vi "TCP Vision - Receiver.vi"() -> ()   [LabVIEW 2019]
doc: "The UDP protocol differs from TCP in that there is no error-checking with the packets of information that are sent, and thus no guarantee whatsoever that an intended recipient will actually receive a given piece of data.\n\nUDP does offer the ability to \"broadcast\" data across a network--simply specify an IP Address of all ones (255.255.255.255) to attempt to broadcast information network-wide. Keep in mind that routers and other network hardware will generally refuse to forward the broadcast beyond certain points, so the extent of the broadcast will in practice be limited."
uses:
  UDP Main States.ctl
  <vilib>/vision/Image Controls.llb/IMAQ Image.ctl
panel:
  in  "receiver port":u16=1180
  out "Image":T1(plugin-control)
  out "error out":errorcluster
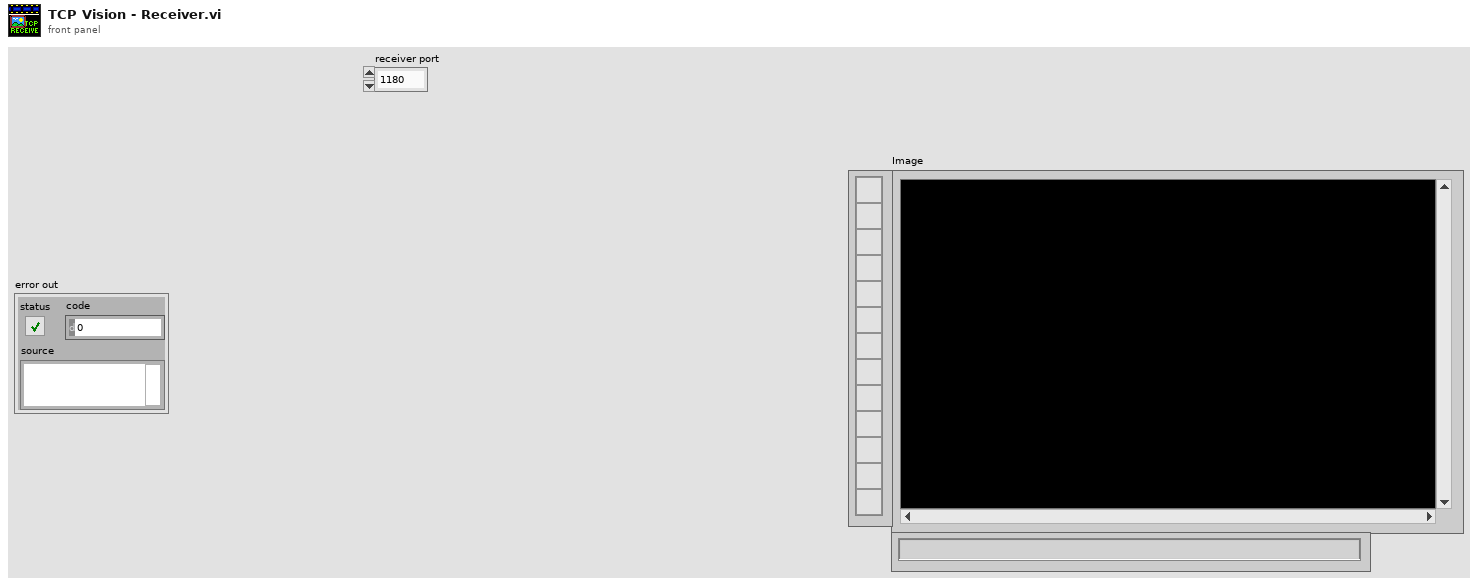
[diagram p1: front panel]
types:
  T1 = typedef "IMAQ Image.ctl" = refnum<image>
  T2 = typedef "UDP Main States.ctl" = enum16{"Message Dispatcher", "INI", "Read Data", "Send Data", "TCP Close", "TCP Open", "Exit"}
  T3 = enum16{"Standard", "Buffered", "CRLF", "Immediate"}
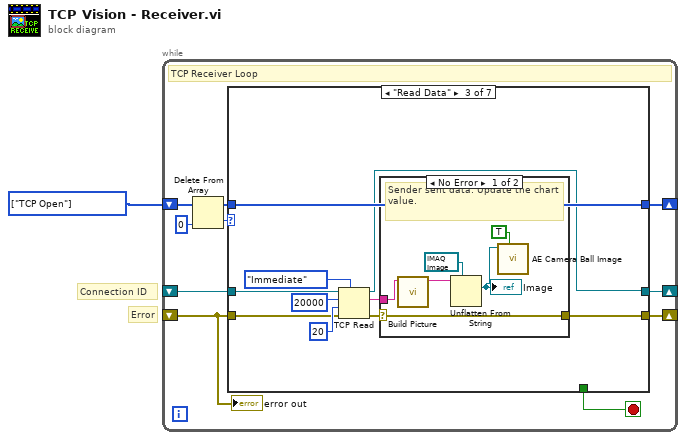
[diagram p0: block diagram]
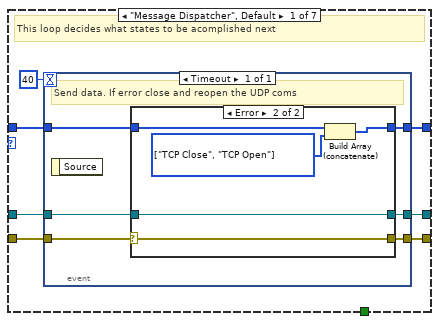
[diagram p2: hidden frame]
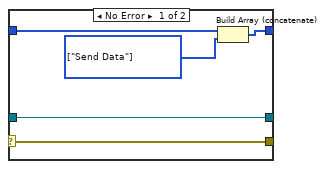
[diagram p3: hidden frame]
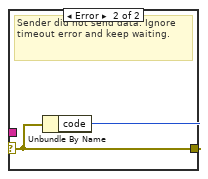
[diagram p5: hidden frame]
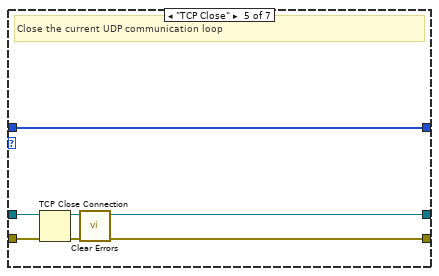
[diagram p8: hidden frame]
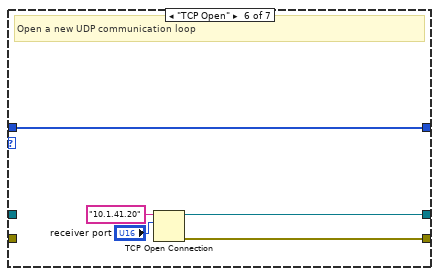
[diagram p9: hidden frame]
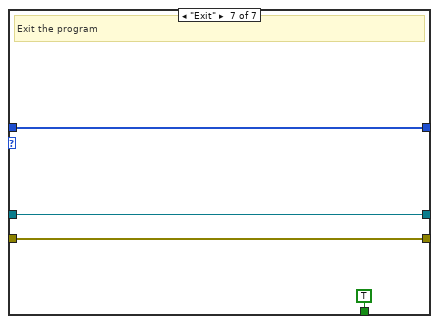
[diagram p10: hidden frame]
diagram:
  w1 = T2[] [enum."TCP Open"] items=["Message Dispatcher", "INI", "Read Data", "Send Data", "TCP Close", "TCP Open", "Exit"]
  # "Error"
  # "Connection ID"
  n1 = while {
    shift-right: [w3] -> _
    shift-left: w1 -> [w7]
    shift-right: [w11] -> _
    shift-left: _ -> [w9]
    shift-right: [w10] -> _
    shift-left: _ -> [w8]
    stop <- w2 stop-if-true
    # "TCP Receiver Loop"
    n2 = Delete From Array(array=w7, index=0) -> (deleted portion=w5:T2, array with subset deleted=w4:T2[])  [unwired: 1 in]
    n3 = case shown="\"Read Data\"" w5 {
      tunnel: [w15 w37 w40 w60 w62 w69 w76] -> w11
      tunnel: [w13 w36 w38 w59 w63 w68 w75] -> w10
      tunnel: w9 -> [w16 w37 w41 w60 w66 _ w76]
      tunnel: w8 -> [w14 w36 w39 w59 w65 _ w75]
      tunnel: w4 -> [w18 w35 w47 w61 w67 w72 w74]
      tunnel: [w17 w35 w47 w61 w67 w72 w74] -> w3
      tunnel: [_ _ _ _ _ _ TRUE] -> w2
      frame "Message Dispatcher", Default {
        # "This loop decides what states to be acomplished next"
        n4 = event shown="[0] Timeout" {
          selector: _ -> [_]
          dyn-events: _ -> [_]
          timeout: 40 -> [_]
          tunnel: w18 -> [w22]
          tunnel: [w21] -> w17
          tunnel: w16 -> [w20]
          tunnel: [w19] -> w15
          tunnel: w14 -> [w24]
          tunnel: [w23] -> w13
          event Timeout {
            # "Send data. If error close and reopen the UDP coms"
            n5 = event-data() -> ()  [unwired: 1 in, 1 out]
            n6 = case shown="Error" w24 {
              selector: w24 -> [w29 w34]
              tunnel: [w29 w34] -> w23
              tunnel: w22 -> [w28 w33]
              tunnel: [w26 w31] -> w21
              tunnel: w20 -> [w27 w32]
              tunnel: [w27 w32] -> w19
              frame No Error {
                w25 = T2[] [enum."Send Data"] items=["Message Dispatcher", "INI", "Read Data", "Send Data", "TCP Close", "TCP Open", "Exit"]
                n7 = Build Array (concatenate)(w28, w25) -> (w26:T2[])
              }
              frame Error {
                w30 = T2[] [enum."TCP Close", enum."TCP Open"] items=["Message Dispatcher", "INI", "Read Data", "Send Data", "TCP Close", "TCP Open", "Exit"]
                n8 = Build Array (concatenate)(w33, w30) -> (w31:T2[])
              }
            }
          }
        }
      }
      frame "INI" {
      }
      frame "Read Data" {
        n9 = TCP Read(connection ID=w41, bytes to read=20000, error in (no error)=w39, 7:T3."Immediate" ("mode (standard)"), 9:20 ("timeout ms (25000)")) -> (connection ID out=w40:refnum<k5>, data out=w45:string, error out=w44:errorcluster)
        n10 = case shown="No Error" w44 {
          selector: w44 -> [w53 w55]
          tunnel: w45 -> [w51 _]
          tunnel: [w53 w54] -> w38
          frame No Error {
            # "Sender sent data. Update the chart value."
            n11 = call "Build Picture.vi"("data string"=w51) -> ("Last Image"=w50:string)  [unwired: 10 in]
            n12 = Unflatten From String(type=T1 refnum ("Image Out"), binary string=w50) -> (value=w49:T1)  [unwired: 3 in, 2 out]
            "Image" <- w49
            n13 = call "AE Camera Ball Image.vi"("Update"=TRUE, "Ball Image in"=w49) -> ()  [unwired: 9 in, 1 out]
          }
          frame Error {
            # "Sender did not send data. Ignore timeout error and keep waiting."
            n14 = Unbundle By Name(w55) -> ("code"=w56:i32)
            n15 = case shown="56" w56 {
              tunnel: w55 -> [w57 _]
              tunnel: [w57 w58] -> w54
              frame Default {
              }
              frame 56 {
                w58 = errorcluster {"status"=FALSE, "code"=0, "source"=""}  # No error
              }
            }
          }
        }
      }
      frame "Send Data" {
        # "Sends camera images to the dashboard"
      }
      frame "TCP Close" {
        # "Close the current UDP communication loop"
        n16 = TCP Close Connection(connection ID=w66, error in (no error)=w65) -> (connection ID out=w62:refnum<k5>, error out=w64:errorcluster)  [unwired: 1 in]
        n17 = call <vilib>:"Clear Errors.vi"("error in (no error)"=w64) -> ("error out"=w63:errorcluster)  [unwired: 5 in, 1 out]
      }
      frame "TCP Open" {
        # "Open a new UDP communication loop"
        n18 = TCP Open Connection(address="10.1.41.20", remote port or service name="receiver port") -> (connection ID=w69:refnum<k5>, error out=w68:errorcluster)  [unwired: 3 in]
      }
      frame "Exit" {
        # "Exit the program"
      }
    }
    "error out" <- w8
  }
